vi "Camera_Snap.vi"(8 "error in (no error)":errorcluster, 10 "Camera Session In":T1, 11 "Image In":T2) -> (0 "error out":errorcluster, 3 "New Image":T2)   [LabVIEW 2019]
uses:
  <vilib>/vision/Image Controls.llb/IMAQ Image.ctl
  <vilib>/userdefined/High Color/IMAQdx.ctl
  <vilib>/vision/driver/NI_Vision_Acquisition_Software.lvlib
panel:
  in  "CameraName":refnum<vi>
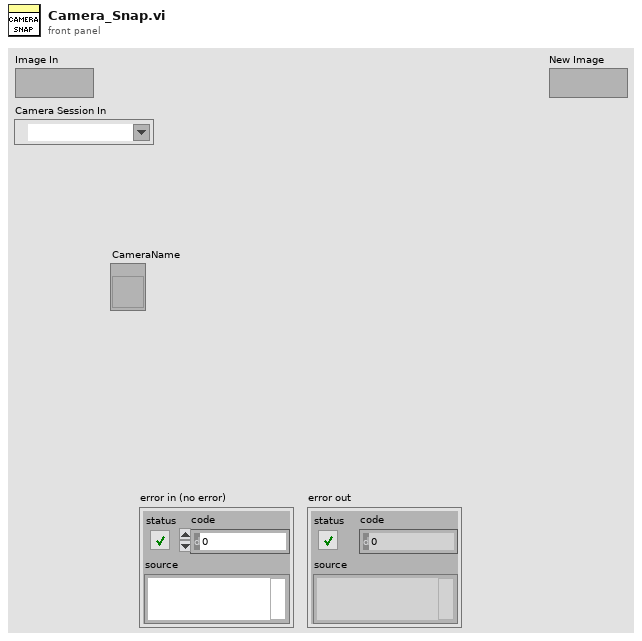
[diagram p1: front panel]
types:
  T1 = typedef "IMAQdx.ctl" = refnum<k21>
  T2 = typedef "IMAQ Image.ctl" = refnum<image>
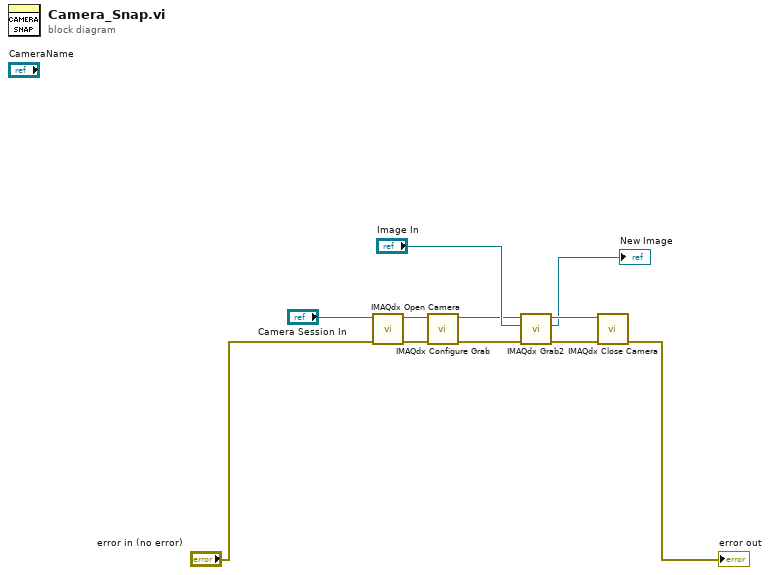
[diagram p0: block diagram]
diagram:
  n1 = call <vilib>:"IMAQdx Open Camera.vi"("error in"="error in (no error)", "Session In"="Camera Session In") -> ("error out"=w7:errorcluster, "Session Out"=w9:T1)  [unwired: 1 in, 7 out]
  n2 = call <vilib>:"IMAQdx Configure Grab.vi"("Session In"=w9) -> ("Session Out"=w2:T1)  [unwired: 9 in, 1 out]
  n3 = call <vilib>:"IMAQdx Grab2.vi"("error in"=w7, "Image In"="Image In", "Session In"=w2) -> ("error out"=w8:errorcluster, "Image Out"=→"New Image":T2, "Session Out"=w10:T1)  [unwired: 5 in, 1 out]
  n4 = call <vilib>:"IMAQdx Close Camera.vi"("error in"=w8, "Session In"=w10) -> ("error out"=→"error out":errorcluster)  [unwired: 9 out]
